vi "Test Initialize Integration.vi"() -> ()   [LabVIEW 2019]
uses:
  Maui 2.0/Maui 2.0.lvclass
  <vilib>/JKI/JKI SMO/SMO/SMO.lvclass
  C:/Program Files (x86)/National Instruments/LabVIEW 2019/vi.lib/JKI/JKI SMO/SMO/SMO.lvclass
  <vilib>/addons/_JKI Toolkits/Caraya/classes/Assert/Assert.lvclass
  <vilib>/addons/_JKI Toolkits/Caraya/classes/Test/Test.lvclass
  <vilib>/addons/_JKI Toolkits/Caraya/classes/Assert/Assert Equal Value_Variant.vi
  Helper/Test Helper 1/Test Helper 1.lvclass
panel:
  out "error out":errorcluster
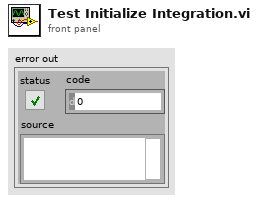
[diagram p1: front panel]
types:
  T1 = cluster{"Control":refnum<vi>, "Subpanel":refnum<vi>, "Active":i32, "Ctrl Class":string}[]
  T2 = cluster{"Control":refnum<vi>, "SubPnl":refnum<vi>}
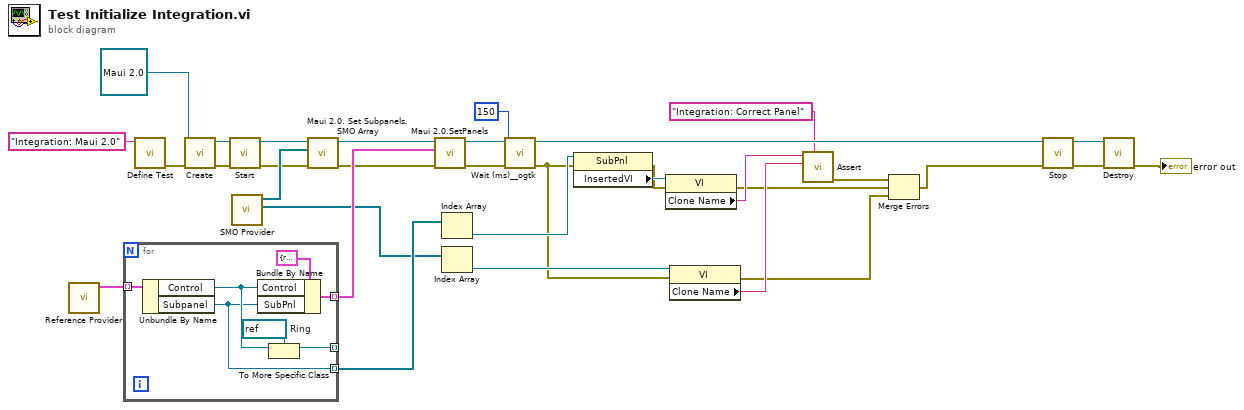
[diagram p0: block diagram]
diagram:
  n1 = call "Reference Provider.vi"() -> ("References"=w25:T1)  [unwired: 11 in]
  n2 = for {
    tunnel: w25 -> [w38] mode=indexing
    tunnel: [w37] -> w24 mode=indexing
    tunnel: [w34] -> _ mode=indexing
    tunnel: [w33] -> w18 mode=indexing
    w36 = refnum<vi> refnum  # Ring
    n3 = Unbundle By Name(w38) -> ("Control"=w35:refnum<vi>, "Subpanel"=w33:refnum<vi>)
    n4 = Bundle By Name(cluster=T2 {"Control"=refnum, "SubPnl"=refnum} ("Panel"), "Control"=w35, "SubPnl"=w33) -> (w37:T2)
    n5 = To More Specific Class(target class=w36, reference=w35) -> (specific class reference=w34:refnum<vi>)  [unwired: 1 in, 1 out]
  }
  n6 = call <vilib>:"Define Test.vi"("Label (VI Title)"="Integration: Maui 2.0") -> ("error out"=w11:errorcluster)  [unwired: 10 in]
  n7 = call <vilib>:"Create.vi"("error in (no error)"=w11, "SMO"=refnum<class "Maui 2.0.lvclass"> refnum ("Maui 2.0.lvclass")) -> ("error out"=w21:errorcluster, "SMO out"=w32:refnum<class "Maui 2.0.lvclass">)  [unwired: 7 in, 1 out]
  n8 = call <vilib>:"Start.vi"("error in (no error)"=w21, "SMO"=w32) -> ("error out"=w22:errorcluster, "SMO out"=w29:refnum<class "Maui 2.0.lvclass">)  [unwired: 8 in]
  n9 = call "SMO Provider.vi"() -> ("Refs"=w17:refnum<vi>[], "SMOs"=w28:refnum<class "Test Helper 1.lvclass">[])  [unwired: 10 in]
  n10 = call-dynamic "Maui 2.0. Set Subpanels.SMO Array.vi"("error in (no error)"=w22, "Subpanels in"=w28, "Maui 2.0 in"=w29) -> ("error out"=w23:errorcluster, "Maui 2.0 out"=w27:refnum<class "Maui 2.0.lvclass">)  [unwired: 6 in, 1 out]
  n11 = call "Maui 2.0.SetPanels.vi"("error in (no error)"=w23, "Set Panels"=w24, "Maui 2.0"=w27) -> ("error out"=w20:errorcluster, "Maui 2.0 out"=w26:refnum<class "Maui 2.0.lvclass">)  [unwired: 7 in]
  n12 = Index Array(array=w18) -> (element=w19:refnum<vi>)  [unwired: 1 in]
  n13 = Index Array(array=w17) -> (element=w14:refnum<vi>)  [unwired: 1 in]
  n14 = call <userlib>:"Wait (ms)__ogtk.vi"("error in (no error)"=w20, "milliseconds to wait"=u32 150) -> ("error out"=w9:errorcluster)  [unwired: 8 in, 1 out]
  n15 = property class="SubPnl"(reference=w19, error in=w9) -> (error out=w8:errorcluster, "InsertedVI"=w16:refnum<vi>)  [unwired: 1 out]
  n16 = property class="VI"(reference=w16, error in=w8) -> (error out=w5:errorcluster, "Clone Name"=w7:string)  [unwired: 1 out]
  n17 = property class="VI"(reference=w14, error in=w9) -> (error out=w4:errorcluster, "Clone Name"=w13:string)  [unwired: 1 out]
  n18 = call-poly <vilib>:"Assert.vi"("Label"="Integration: Correct Panel", "Y"=w13, "X"=w7) -> ("error out"=w6:errorcluster)  [unwired: 8 in]
  n19 = Merge Errors(w6, w5, w4) -> (w3:errorcluster)
  n20 = call <vilib>:"Stop.vi"("error in (no error)"=w3, "SMO"=w26) -> ("error out"=w2:errorcluster, "SMO out"=w31:refnum<class "Maui 2.0.lvclass">)  [unwired: 8 in]
  n21 = call <vilib>:"Destroy.vi"("error in (no error)"=w2, "SMO"=w31) -> ("error out"=→"error out":errorcluster)  [unwired: 9 in]
